vi "Start.vi"(6 "Transport":refnum<class "Transport.lvclass">, 7 "Actor in":refnum<class "Actor.lvclass">, 9 "Actor Ref":refnum<vi>, 10 "Spawn":refnum<class "Spawn.lvclass">) -> (0 "Error out":errorcluster, 5 "Actor out":refnum<class "Actor.lvclass">)   [LabVIEW 2025, in "jettl.lvlib"]
uses:
  jettl.lvlib
  Teardown Location.ctl
  Msg/Msg.lvclass
  Msg Set.ctl
  Attributes/Attributes/Attributes.lvclass
  Setup.ctl
  Transport/Transport/Transport.lvclass
  Setup/Setup.lvlib
  Spawn/Spawn/Spawn.lvclass
  Actor/Actor.lvclass
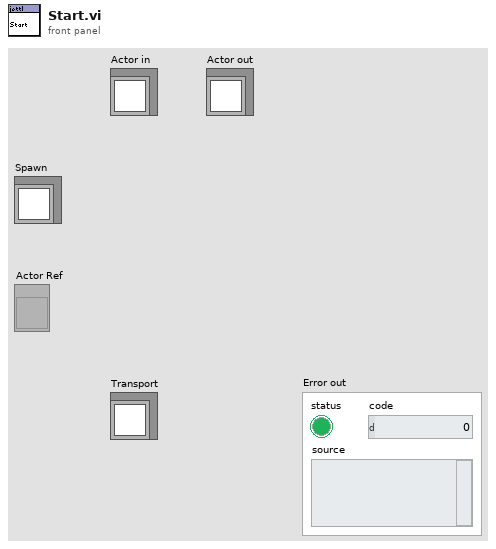
[diagram p1: front panel]
types:
  T1 = typedef "jettl.lvlib/Setup.ctl" = cluster{"Unified Msg Set":T2, "UID":string, "Parent Attributes":refnum<class "Attributes.lvclass">, "Queue of Self Attributes":refnum<queue>, "Actor Ref":refnum<vi>, "Transport":refnum<class "Transport.lvclass">}
  T2 = typedef "jettl.lvlib/Msg Set.ctl" = set{refnum<class "Msg.lvclass">}
  T3 = typedef "jettl.lvlib/Teardown Location.ctl" = enum16{"Start", "Stop"}
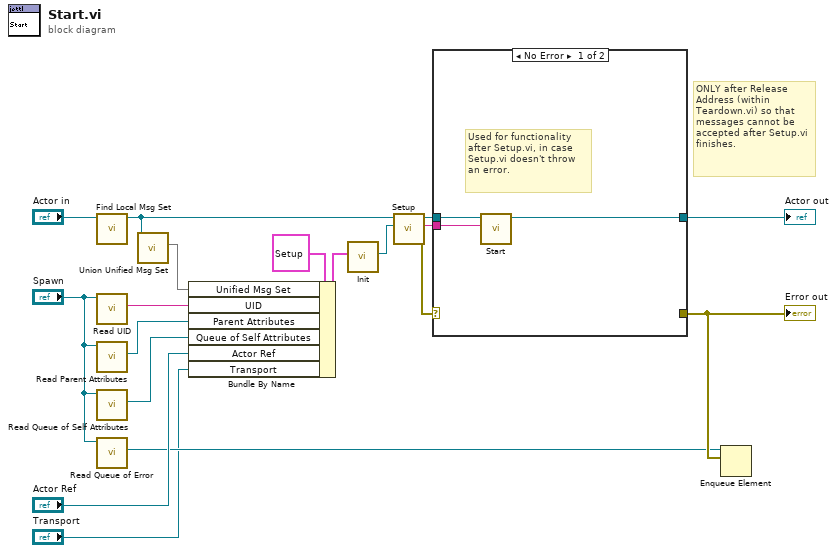
[diagram p0: block diagram]
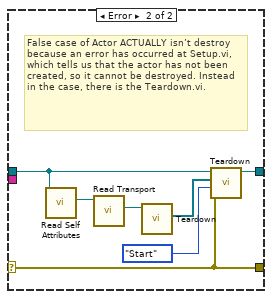
[diagram p2: hidden frame]
diagram:
  # "ONLY after Release Address (within Teardown.vi) so that messages cannot be accepted after Setup.vi finishes."
  n1 = call-dynamic "Find Local Msg Set.vi"("Actor in"="Actor in") -> ("Actor out"=w17:refnum<class "Actor.lvclass">)  [unwired: 10 in]
  n2 = call-dynamic "Read UID.vi"("Spawn in"="Spawn") -> ("UID"=w6:string)  [unwired: 10 in]
  n3 = call-dynamic "Read Parent Attributes.vi"("Spawn in"="Spawn") -> ("Parent Attributes"=w5:refnum<class "Attributes.lvclass">)  [unwired: 10 in]
  n4 = call-dynamic "Read Queue of Self Attributes.vi"("Spawn in"="Spawn") -> ("Queue of Self Attributes"=w4:refnum<queue>)  [unwired: 10 in]
  n5 = call-dynamic "Read Queue of Error.vi"("Spawn in"="Spawn") -> ("Queue of Error"=w3:refnum<queue>)  [unwired: 10 in]
  n6 = call-dynamic "Union Unified Msg Set.vi"("Get Actor in"=w17) -> ("Unified Msg Set"=w11:T2)  [unwired: 10 in]
  n7 = Bundle By Name(cluster=T1 {"Unified Msg Set"={}, "UID"="", "Parent Attributes"=refnum, "Queue of Self Attributes"=refnum, "Actor Ref"=refnum, "Transport"=refnum} ("Setup"), "Unified Msg Set"=w11, "UID"=w6, "Parent Attributes"=w5, "Queue of Self Attributes"=w4, "Actor Ref"="Actor Ref", "Transport"="Transport") -> (w9:T1)
  n8 = call "Init.vi"("Setup"=w9) -> ("Setup"=w8:refnum<class "Setup.lvclass">)  [unwired: 10 in]
  n9 = call-dynamic "Setup.vi"("Setup"=w8, "Actor in"=w17) -> ("Error out"=w14:errorcluster, "Setup Output"=w1:string, "Actor out"=w16:refnum<class "Actor.lvclass">)  [unwired: 7 in]
  n10 = case shown="No Error" w14 {
    selector: w14 -> [_ w27]
    tunnel: w16 -> [w21 w24]
    tunnel: [_ w27] -> w13
    tunnel: [w20 w28] -> w15
    tunnel: w1 -> [w19 _]
    frame No Error {
      # "Used for functionality after Setup.vi, in case Setup.vi doesn't throw an error."
      n11 = call-dynamic "Start.vi"("Setup Output"=w19, "Actor in"=w21) -> ("Actor out"=w20:refnum<class "Actor.lvclass">)  [unwired: 9 in]
    }
    frame Error {
      # "False case of Actor ACTUALLY isn’t destroy because an error has occurred at Setup.vi, which tells us that the actor has not been created, so it cannot be destroyed. Instead in the case, there is the Teardown.vi."
      n12 = call-dynamic "Read Self Attributes.vi"("Actor in"=w24) -> ("Self Attributes"=w23:refnum<class "Attributes.lvclass">)  [unwired: 10 in]
      n13 = call-dynamic "Read Transport.vi"("Attributes in"=w23) -> ("Transport"=w22:refnum<class "Transport.lvclass">)  [unwired: 10 in]
      n14 = call-dynamic "Teardown.vi"("Transport in"=w22) -> ("Unhandled Msgs"=w25:refnum<class "Msg.lvclass">[])  [unwired: 10 in]
      n15 = call-dynamic "Teardown.vi"("Error in"=w27, "Teardown Location"=Teardown_Location."Start", "Unhandled Msgs"=w25, "Actor in"=w24) -> ("Actor out"=w28:refnum<class "Actor.lvclass">)  [unwired: 7 in]
    }
  }
  "Actor out" <- w15
  "Error out" <- w13
  n16 = Enqueue Element(queue=w3, element=w13) -> ()  [unwired: 2 in, 3 out]
